vi "scheme-probe.vi"(11 "Material-Scheme.lvclass":refnum<class "Material-Scheme.lvclass">) -> (2 "Value String":string, 3 "Boolean":bool)   [LabVIEW 2021, in "TSC Material Theme.lvlib" / "Material-Scheme.lvclass"]
uses:
  Material-Scheme.lvclass
  Material-Scheme.lvclass/Material-Scheme.ctl
panel:
  out "Scrim":u32(colorbox)
  out "Shadow":u32(colorbox)
  out "Inverse Primary":u32(colorbox)
  out "Inverse on Surface":u32(colorbox)
  out "Inverse Surface":u32(colorbox)
  out "On Error Container":u32(colorbox)
  out "Error Container":u32(colorbox)
  out "On Error":u32(colorbox)
  out "Error":u32(colorbox)
  out "Outline":u32(colorbox)
  out "Outline Variant":u32(colorbox)
  out "On Surface Var":u32(colorbox)
  out "On Surface":u32(colorbox)
  out "Surf Container Highest":u32(colorbox)
  out "Surf Container":u32(colorbox)
  out "Surf Container High":u32(colorbox)
  out "Surf Container Low":u32(colorbox)
  out "Surf Container Lowest":u32(colorbox)
  out "Surface Bright":u32(colorbox)
  out "Surface":u32(colorbox)
  out "Surface Dim":u32(colorbox)
  out "Tertiary Fixed":u32(colorbox)
  out "On Tertiary Fixed Variant":u32(colorbox)
  out "On Tertiary Fixed":u32(colorbox)
  out "Tertiary Fixed\nDim":u32(colorbox)
  out "On Tertiary Container":u32(colorbox)
  out "Tertiary Container":u32(colorbox)
  out "On Tertiary":u32(colorbox)
  out "Tertiary":u32(colorbox)
  out "Secondary\nFixed":u32(colorbox)
  out "On Secondary Fixed Variant":u32(colorbox)
  out "On Secondary Fixed":u32(colorbox)
  out "Secondary\nFixed Dim":u32(colorbox)
  out "On Secondary Container":u32(colorbox)
  out "Secondary Container":u32(colorbox)
  out "On Secondary":u32(colorbox)
  out "Secondary":u32(colorbox)
  out "On Primary Fixed Variant":u32(colorbox)
  out "On Primary Fixed":u32(colorbox)
  out "Primary Fixed\nDim":u32(colorbox)
  out "Primary Fixed":u32(colorbox)
  out "On Primary Container":u32(colorbox)
  out "Primary Container":u32(colorbox)
  out "On Primary":u32(colorbox)
  out "Primary":u32(colorbox)
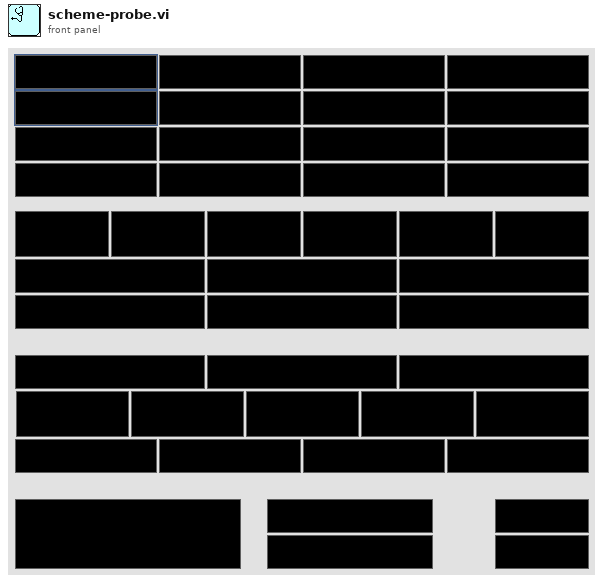
[diagram p1: front panel]
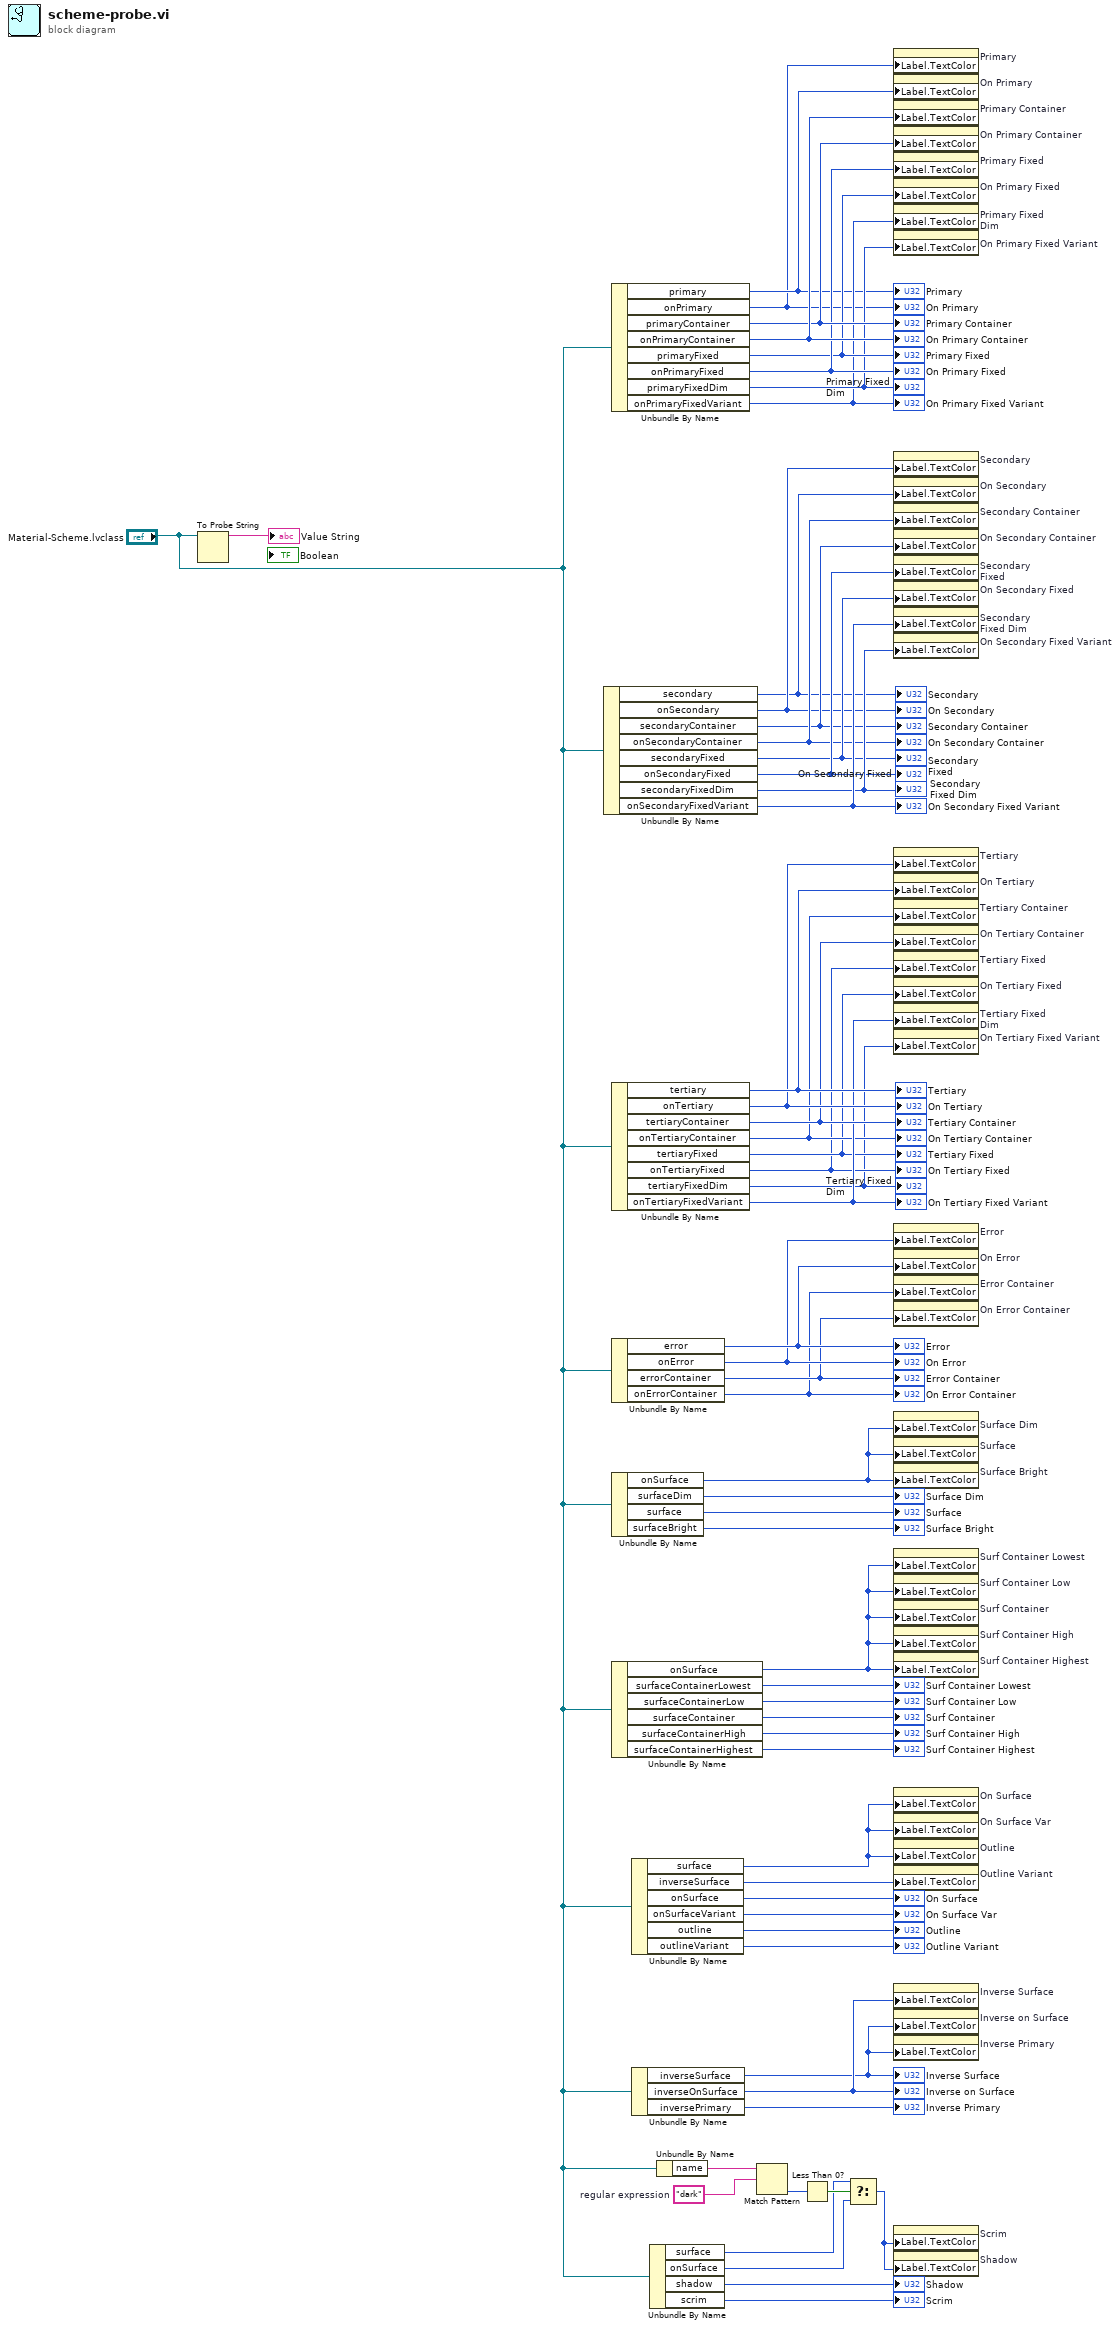
[diagram p0: block diagram]
diagram:
  w9 = "dark"  # regular expression
  n1 = To Probe String(7:"Material-Scheme.lvclass") -> (3:→"Value String":string)  [unwired: 2 in, 1 out]
  n2 = Unbundle By Name("Material-Scheme.lvclass") -> ("secondary"=w44:u32, "onSecondary"=w45:u32, "secondaryContainer"=w46:u32, "onSecondaryContainer"=w47:u32, "secondaryFixed"=w48:u32, "onSecondaryFixed"=w49:u32, "secondaryFixedDim"=w50:u32, "onSecondaryFixedVariant"=w51:u32)
  "Secondary" <- w44
  "On Secondary" <- w45
  "Secondary Container" <- w46
  "On Secondary Container" <- w47
  "Secondary\nFixed Dim" <- w50
  "On Secondary Fixed" <- w49
  "On Secondary Fixed Variant" <- w51
  "Secondary\nFixed" <- w48
  n3 = Unbundle By Name("Material-Scheme.lvclass") -> ("primary"=w3:u32, "onPrimary"=w2:u32, "primaryContainer"=w56:u32, "onPrimaryContainer"=w57:u32, "primaryFixed"=w54:u32, "onPrimaryFixed"=w55:u32, "primaryFixedDim"=w53:u32, "onPrimaryFixedVariant"=w52:u32)
  "Primary" <- w3
  "On Primary" <- w2
  "Primary Container" <- w56
  "On Primary Container" <- w57
  "Primary Fixed" <- w54
  "Primary Fixed\nDim" <- w53
  "On Primary Fixed" <- w55
  "On Primary Fixed Variant" <- w52
  n4 = Unbundle By Name("Material-Scheme.lvclass") -> ("tertiary"=w43:u32, "onTertiary"=w42:u32, "tertiaryContainer"=w41:u32, "onTertiaryContainer"=w39:u32, "tertiaryFixed"=w38:u32, "onTertiaryFixed"=w37:u32, "tertiaryFixedDim"=w36:u32, "onTertiaryFixedVariant"=w40:u32)
  "Tertiary" <- w43
  "On Tertiary" <- w42
  "Tertiary Container" <- w41
  "On Tertiary Container" <- w39
  "Tertiary Fixed\nDim" <- w36
  "On Tertiary Fixed" <- w37
  "On Tertiary Fixed Variant" <- w40
  "Tertiary Fixed" <- w38
  n5 = Unbundle By Name("Material-Scheme.lvclass") -> ("error"=w35:u32, "onError"=w34:u32, "errorContainer"=w33:u32, "onErrorContainer"=w32:u32)
  "Error" <- w35
  "On Error" <- w34
  "Error Container" <- w33
  "On Error Container" <- w32
  n6 = Unbundle By Name("Material-Scheme.lvclass") -> ("onSurface"=w28:u32, "surfaceDim"=→"Surface Dim":u32, "surface"=→"Surface":u32, "surfaceBright"=→"Surface Bright":u32)
  n7 = Unbundle By Name("Material-Scheme.lvclass") -> ("onSurface"=w22:u32, "surfaceContainerLowest"=→"Surf Container Lowest":u32, "surfaceContainerLow"=→"Surf Container Low":u32, "surfaceContainer"=→"Surf Container":u32, "surfaceContainerHigh"=→"Surf Container High":u32, "surfaceContainerHighest"=→"Surf Container Highest":u32)
  n8 = Unbundle By Name("Material-Scheme.lvclass") -> ("surface"=w17:u32, "inverseSurface"=w16:u32, "onSurface"=→"On Surface":u32, "onSurfaceVariant"=→"On Surface Var":u32, "outline"=→"Outline":u32, "outlineVariant"=→"Outline Variant":u32)
  n9 = Unbundle By Name("Material-Scheme.lvclass") -> ("inverseSurface"=w13:u32, "inverseOnSurface"=w14:u32, "inversePrimary"=→"Inverse Primary":u32)
  "Inverse Surface" <- w13
  "Inverse on Surface" <- w14
  n10 = Unbundle By Name("Material-Scheme.lvclass") -> ("surface"=w6:u32, "onSurface"=w5:u32, "shadow"=→"Shadow":u32, "scrim"=→"Scrim":u32)
  n11 = Unbundle By Name("Material-Scheme.lvclass") -> ("name"=w10:string)
  n12 = Match Pattern(string=w10, regular expression=w9) -> (offset past match=w8:i32)  [unwired: 1 in, 3 out]
  n13 = Less Than 0?(x=w8) -> (x < 0?=w7:bool)
  n14 = Select(t=w6, s=w7, f=w5) -> (s? t:f=w4:u32)
  n15 = property on="Primary" class="ColBox"("Label.TextColor"=w2) -> ()  [unwired: 2 in, 2 out]
  n16 = property on="On Primary" class="ColBox"("Label.TextColor"=w3) -> ()  [unwired: 2 in, 2 out]
  n17 = property on="Primary Container" class="ColBox"("Label.TextColor"=w57) -> ()  [unwired: 2 in, 2 out]
  n18 = property on="On Primary Container" class="ColBox"("Label.TextColor"=w56) -> ()  [unwired: 2 in, 2 out]
  n19 = property on="Primary Fixed" class="ColBox"("Label.TextColor"=w55) -> ()  [unwired: 2 in, 2 out]
  n20 = property on="On Primary Fixed" class="ColBox"("Label.TextColor"=w54) -> ()  [unwired: 2 in, 2 out]
  n21 = property on="Primary Fixed\nDim" class="ColBox"("Label.TextColor"=w52) -> ()  [unwired: 2 in, 2 out]
  n22 = property on="On Primary Fixed Variant" class="ColBox"("Label.TextColor"=w53) -> ()  [unwired: 2 in, 2 out]
  n23 = property on="Secondary" class="ColBox"("Label.TextColor"=w45) -> ()  [unwired: 2 in, 2 out]
  n24 = property on="On Secondary" class="ColBox"("Label.TextColor"=w44) -> ()  [unwired: 2 in, 2 out]
  n25 = property on="Secondary Container" class="ColBox"("Label.TextColor"=w47) -> ()  [unwired: 2 in, 2 out]
  n26 = property on="On Secondary Container" class="ColBox"("Label.TextColor"=w46) -> ()  [unwired: 2 in, 2 out]
  n27 = property on="Secondary\nFixed" class="ColBox"("Label.TextColor"=w49) -> ()  [unwired: 2 in, 2 out]
  n28 = property on="On Secondary Fixed" class="ColBox"("Label.TextColor"=w48) -> ()  [unwired: 2 in, 2 out]
  n29 = property on="Secondary\nFixed Dim" class="ColBox"("Label.TextColor"=w51) -> ()  [unwired: 2 in, 2 out]
  n30 = property on="On Secondary Fixed Variant" class="ColBox"("Label.TextColor"=w50) -> ()  [unwired: 2 in, 2 out]
  n31 = property on="Tertiary" class="ColBox"("Label.TextColor"=w42) -> ()  [unwired: 2 in, 2 out]
  n32 = property on="On Tertiary" class="ColBox"("Label.TextColor"=w43) -> ()  [unwired: 2 in, 2 out]
  n33 = property on="Tertiary Container" class="ColBox"("Label.TextColor"=w39) -> ()  [unwired: 2 in, 2 out]
  n34 = property on="On Tertiary Container" class="ColBox"("Label.TextColor"=w41) -> ()  [unwired: 2 in, 2 out]
  n35 = property on="Tertiary Fixed" class="ColBox"("Label.TextColor"=w37) -> ()  [unwired: 2 in, 2 out]
  n36 = property on="On Tertiary Fixed" class="ColBox"("Label.TextColor"=w38) -> ()  [unwired: 2 in, 2 out]
  n37 = property on="Tertiary Fixed\nDim" class="ColBox"("Label.TextColor"=w40) -> ()  [unwired: 2 in, 2 out]
  n38 = property on="On Tertiary Fixed Variant" class="ColBox"("Label.TextColor"=w36) -> ()  [unwired: 2 in, 2 out]
  n39 = property on="Error" class="ColBox"("Label.TextColor"=w34) -> ()  [unwired: 2 in, 2 out]
  n40 = property on="On Error" class="ColBox"("Label.TextColor"=w35) -> ()  [unwired: 2 in, 2 out]
  n41 = property on="Error Container" class="ColBox"("Label.TextColor"=w32) -> ()  [unwired: 2 in, 2 out]
  n42 = property on="On Error Container" class="ColBox"("Label.TextColor"=w33) -> ()  [unwired: 2 in, 2 out]
  n43 = property on="Surface Dim" class="ColBox"("Label.TextColor"=w28) -> ()  [unwired: 2 in, 2 out]
  n44 = property on="Surface" class="ColBox"("Label.TextColor"=w28) -> ()  [unwired: 2 in, 2 out]
  n45 = property on="Surface Bright" class="ColBox"("Label.TextColor"=w28) -> ()  [unwired: 2 in, 2 out]
  n46 = property on="Surf Container Lowest" class="ColBox"("Label.TextColor"=w22) -> ()  [unwired: 2 in, 2 out]
  n47 = property on="Surf Container Low" class="ColBox"("Label.TextColor"=w22) -> ()  [unwired: 2 in, 2 out]
  n48 = property on="Surf Container" class="ColBox"("Label.TextColor"=w22) -> ()  [unwired: 2 in, 2 out]
  n49 = property on="Surf Container High" class="ColBox"("Label.TextColor"=w22) -> ()  [unwired: 2 in, 2 out]
  n50 = property on="Surf Container Highest" class="ColBox"("Label.TextColor"=w22) -> ()  [unwired: 2 in, 2 out]
  n51 = property on="On Surface" class="ColBox"("Label.TextColor"=w17) -> ()  [unwired: 2 in, 2 out]
  n52 = property on="On Surface Var" class="ColBox"("Label.TextColor"=w17) -> ()  [unwired: 2 in, 2 out]
  n53 = property on="Outline" class="ColBox"("Label.TextColor"=w17) -> ()  [unwired: 2 in, 2 out]
  n54 = property on="Outline Variant" class="ColBox"("Label.TextColor"=w16) -> ()  [unwired: 2 in, 2 out]
  n55 = property on="Inverse Surface" class="ColBox"("Label.TextColor"=w14) -> ()  [unwired: 2 in, 2 out]
  n56 = property on="Inverse on Surface" class="ColBox"("Label.TextColor"=w13) -> ()  [unwired: 2 in, 2 out]
  n57 = property on="Inverse Primary" class="ColBox"("Label.TextColor"=w13) -> ()  [unwired: 2 in, 2 out]
  n58 = property on="Scrim" class="ColBox"("Label.TextColor"=w4) -> ()  [unwired: 2 in, 2 out]
  n59 = property on="Shadow" class="ColBox"("Label.TextColor"=w4) -> ()  [unwired: 2 in, 2 out]
